vi "GV_undo.vi"(8 "error in (no error)":errorcluster, 9 "Coords":T1, 11 "Gviewer in":refnum<class "Gviewer.lvclass">) -> (0 "error out":errorcluster, 3 "Gviewer out":refnum<class "Gviewer.lvclass">)   [LabVIEW 2020, in "Sgraph_lib_V1.lvlib" / "Gviewer.lvclass"]
doc: "Perform a pan/zoom undo action"
uses:
  Gviewer.lvclass
  <vilib>/Utility/miscctls.llb/LVPoint32TypeDef.ctl
  Gviewer.lvclass/Gviewer.ctl
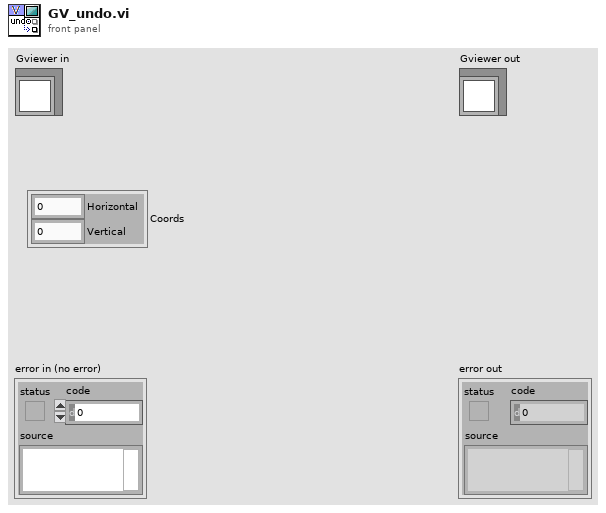
[diagram p1: front panel]
types:
  T1 = typedef "LVPoint32TypeDef.ctl" = cluster{"Horizontal":i32, "Vertical":i32}
  T2 = typedef "Sgraph_lib_V1.lvlib/Gviewer.lvclass/Typedef_ZoomEvent.ctl" = cluster{"Time-Start":timestamp, "Time-End":timestamp, "TimeSpan(sec)":dbl, "Live":T3, "SelProperties":T4[], "Time Stamp":timestamp}
  T3 = typedef "Sgraph_lib_V1.lvlib/Gviewer.lvclass/Typedef_Live.ctl" = enum16{"Live View", "Freeze"}
  T4 = typedef "Sgraph_lib_V1.lvlib/Gviewer.lvclass/Typedef_SelProperties.ctl" = cluster{"Color":u32, "LineType":T5, "max":dbl, "min":dbl, "unit":string}
  T5 = typedef "Sgraph_lib_V1.lvlib/Gviewer.lvclass/Typedef_LineType.ctl" = enum16{"num_bare", "num_MinMax_Area", "num_MinMax_Lines", "num_MinMax_Forfor", "num_Max_Area", "num_Max_Line", "num_Max_Forfor", "num_Min_Area", "num_Min_Line", "num_Min_Fosfor", "Boolean_Line_01", "Boolean_Area_01", "Boolean_Fosfor_01", "Boolean_Line_TF", "Boolean_Area_TF", "Boolean_Fosfor_TF", "Boolean_OnOff_Line", "Boolean_OnOff_Area", "Boolean_OnOff_Fosfor", "Boolean_spare", "StringEvent_Line", "StringEvent_TimeLine"}
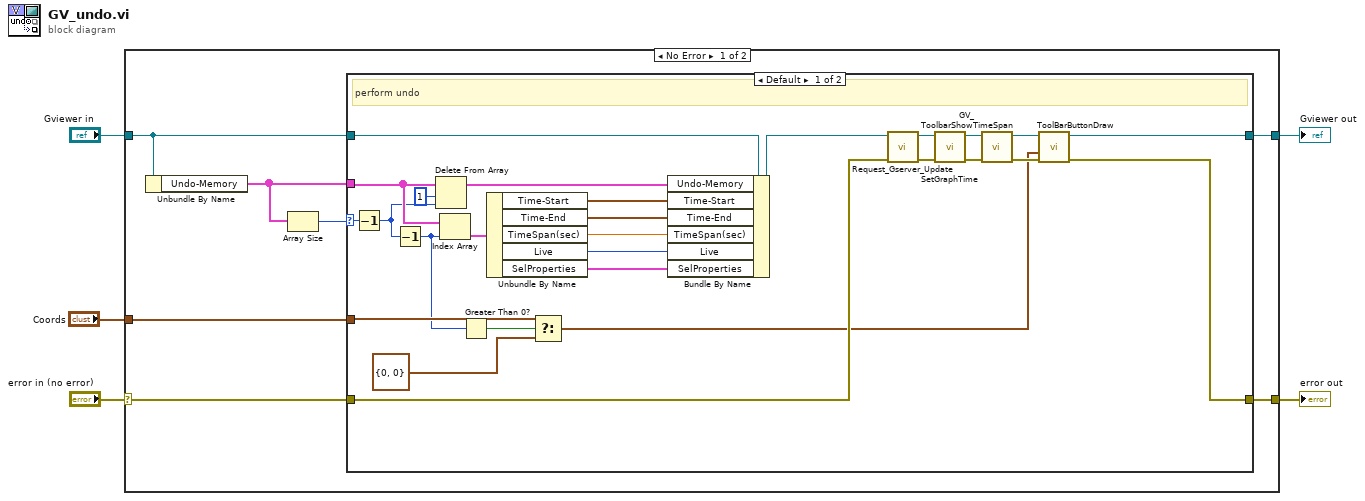
[diagram p0: block diagram]
diagram:
  n1 = case shown="No Error" "error in (no error)" {
    selector: "error in (no error)" -> [w10 w43]
    tunnel: [w9 w43] -> w4
    tunnel: [w8 w42] -> w2
    tunnel: "Gviewer in" -> [w11 w42]
    tunnel: "Coords" -> [w6 _]
    frame No Error {
      n2 = Unbundle By Name(w11) -> ("Undo-Memory"=w7:T2[])
      n3 = Array Size(array=w7) -> (size(s)=w12:i32)
      n4 = case shown="Default" w12 {
        selector: w12 -> [w39 _]
        tunnel: w11 -> [w36 w40]
        tunnel: w10 -> [w24 w41]
        tunnel: [w20 w41] -> w9
        tunnel: [w22 w40] -> w8
        tunnel: w7 -> [w15 _]
        tunnel: w6 -> [w19 _]
        frame Default {
          # "perform undo"
          n5 = Decrement(x=w39) -> (x-1=w14:i32)
          n6 = Decrement(x=w14) -> (x-1=w13:i32)
          n7 = Delete From Array(array=w15, length=1, index=w14) -> (array with subset deleted=w37:T2[])  [unwired: 1 out]
          n8 = Index Array(array=w15, index=w13) -> (element=w35:T2)
          n9 = Greater Than 0?(x=w13) -> (x > 0?=w17:bool)
          n10 = Unbundle By Name(w35) -> ("Time-Start"=w34:timestamp, "Time-End"=w33:timestamp, "TimeSpan(sec)"=w32:dbl, "Live"=w31:T3, "SelProperties"=w30:T4[])
          n11 = Select(t=w19, s=w17, f=T1 {"Horizontal"=0, "Vertical"=0}) -> (s? t:f=w16:T1)
          n12 = Bundle By Name(cluster=w36, "Undo-Memory"=w37, "Time-Start"=w34, "Time-End"=w33, "TimeSpan(sec)"=w32, "Live"=w31, "SelProperties"=w30) -> (w25:refnum<class "Gviewer.lvclass">)
          n13 = call "Request_Gserver_Update.vi"("error in (no error)"=w24, "Gviewer in"=w25) -> ("error out"=w28:errorcluster, "Gviewer out"=w29:refnum<class "Gviewer.lvclass">)  [unwired: 8 in]
          n14 = call "SetGraphTime.vi"("error in (no error)"=w28, "Gviewer in"=w29) -> ("error out"=w27:errorcluster, "Gviewer out"=w26:refnum<class "Gviewer.lvclass">)  [unwired: 8 in]
          n15 = call "GV_ToolbarShowTimeSpan.vi"("error in (no error)"=w27, "Gviewer in"=w26) -> ("error out"=w21:errorcluster, "Gviewer out"=w23:refnum<class "Gviewer.lvclass">)  [unwired: 7 in, 1 out]
          n16 = call "ToolBarButtonDraw.vi"("error in (no error)"=w21, "Coords"=w16, "Gviewer in"=w23) -> ("error out"=w20:errorcluster, "Gviewer out"=w22:refnum<class "Gviewer.lvclass">)  [unwired: 7 in]
        }
        frame 0 {
          # "memory empty"
        }
      }
    }
    frame Error {
    }
  }
  "error out" <- w4
  "Gviewer out" <- w2
